vi "Relay Signal (Bool).vi"(4 "User Parameter":T1, 5 "Event Data":cluster{"Bool Value":bool}, 6 "User Event Ref":refnum<user-event>, 7 "Event Common Data":T3 {"Event Source" items=["LabVIEW UI"=0, "ActiveX"=1, "User Event"=25]}) -> ()   [LabVIEW 2013, in "Template.lvlib" / "LQCoreEngine.lvclass"]
uses:
  LQCoreEngine.lvclass
  <vilib>/event_ctls.llb/eventsource.ctl
  Template.lvlib
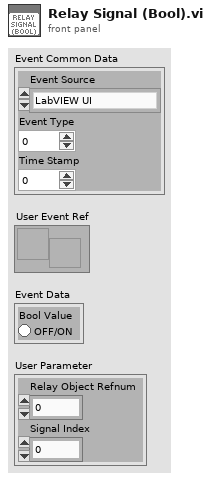
[diagram p1: front panel]
types:
  T1 = cluster{"Relay Object Refnum":u64, "Signal Index":i32}
  T2 = typedef "eventsource.ctl" = u32
  T3 = cluster{"Event Source":T2, "Event Type":u32, "Time Stamp":u32}
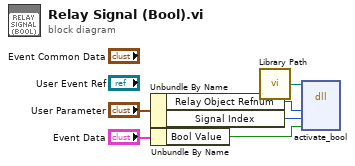
[diagram p0: block diagram]
diagram:
  n1 = Unbundle By Name("User Parameter") -> ("Relay Object Refnum"=w3:u64, "Signal Index"=w4:i32)
  n2 = Unbundle By Name("Event Data") -> ("Bool Value"=w2:bool)
  n3 = call "Library Path.vi"() -> ("Library Path"=w1:path)
  n4 = dll-call lib="?" fn="activate_bool"(path in=w1, "_instance"=w3, "signalIndex"=w4, "data"=w2) -> ()  [unwired: 6 in, 2 out]
